vi "PRINCIPAL.vi"() -> ()   [LabVIEW 2019]
uses:
  <vilib>/Analysis/baseanly.llb/Real Dot Product.vi
  <vilib>/Analysis/baseanly.llb/A x Vector.vi
  <vilib>/addons/control/pid/pid.llb/PID (DBL).vi
  <vilib>/Analysis/NI_AALBase.lvlib
  <vilib>/addons/control/pid/NI_PID_pid.lvlib
panel:
  out "FT":picture
  in  "LAZO CERRADO":bool
  in  "setpoint":dbl format="%.2f"
  out "GRAFICA":cluster{"U(t)":dbl, "Y(t)":dbl, dbl}(graph)
  out "Y(t)":dbl format="%.2f"
  out "U(t)":dbl
  in  "Retardo":dbl min=0.0 format="%#_3g"
  in  "Denominador":dbl[](array[numeric])
  in  "Numerador":dbl[](array[numeric])=[0.0, 2.0, 1.0]
  # "LAZO ABIERTO"
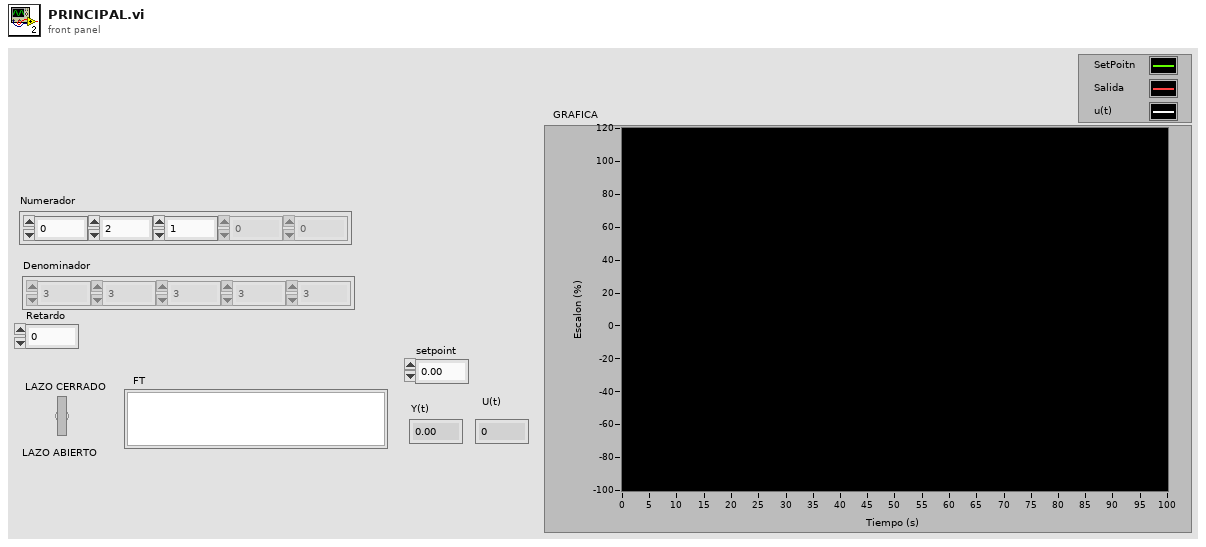
[diagram p1: front panel]
types:
  T1 = typedef "NI_Matrix.lvlib/RealMatrix.ctl" = dbl[][]
  T2 = cluster{"proportional gain (Kc)":dbl, "integral time (Ti, min)":dbl, "derivative time (Td, min)":dbl}
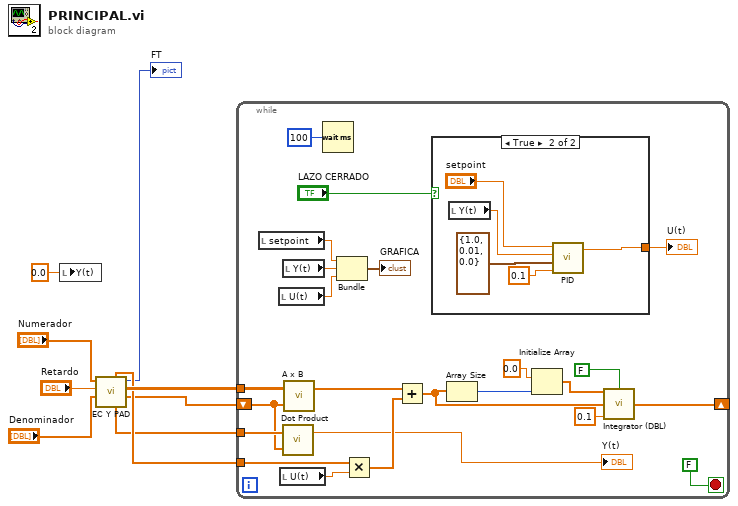
[diagram p0: block diagram]
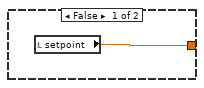
[diagram p2: hidden frame]
diagram:
  n1 = local write "Y(t)"(0.0 ("Y(t)")) -> ()
  n2 = call "EC Y PAD.vi"("Denominador"="Denominador", "Retardo"="Retardo", "Numerador"="Numerador") -> ("Array"=w7:dbl[], "A"=w9:T1, "FT"=→"FT":picture, "C"=w6:dbl[], "B"=w8:dbl[])  [unwired: 4 in]
  n3 = while {
    tunnel: w9 -> [w31]
    tunnel: w8 -> [w30]
    tunnel: w6 -> [w27]
    shift-right: [w19] -> _
    shift-left: w7 -> [w26]
    stop <- FALSE stop-if-true
    n4 = local read "setpoint"() -> (w12:dbl)
    n5 = local read "U(t)"() -> (w15:dbl)
    n6 = local read "U(t)"() -> (w17:dbl)
    n7 = local read "Y(t)"() -> (w13:dbl)
    n8 = call-poly <vilib>:"Dot Product.vi"("Y Vector"=w26, "X Vector"=w27) -> ("X * Y"=→"Y(t)":dbl)  [unwired: 1 out]
    n9 = call-poly <vilib>:"A x B.vi"("Vector"=w26, "A"=w31) -> ("A x Vector"=w29:dbl[])  [unwired: 1 out]
    n10 = Wait (ms)(milliseconds to wait=u32 100) -> ()  [unwired: 1 out]
    n11 = Bundle("setpoint"=w12, "Y(t)"=w13, "U(t)"=w15) -> (→"GRAFICA":cluster{"setpoint":dbl, "Y(t)":dbl, " U(t)":dbl})  [unwired: 1 in]
    n12 = Multiply(x=w30, y=w17) -> (x*y=w28:dbl[])
    n13 = Add ("Add.vi")(x=w29, y=w28) -> (x+y=w23:dbl[])
    n14 = case shown="True" "LAZO CERRADO" {
      tunnel: [w33 w35] -> w11
      frame False {
        n15 = local read "setpoint"() -> (w33:dbl)
      }
      frame True {
        n16 = local read "Y(t)"() -> (w37:dbl)
        n17 = call-poly <vilib>:"PID.vi"("dt (s)"=0.1, "PID gains"=T2 {"proportional gain (Kc)"=1.0, "integral time (Ti, min)"=0.01, "derivative time (Td, min)"=0.0}, "process variable"=w37, "setpoint"="setpoint") -> ("output"=w35:dbl)  [unwired: 6 in, 1 out]
      }
    }
    "U(t)" <- w11
    n18 = Array Size(array=w23) -> (size(s)=w22:i32)
    n19 = Initialize Array(0.0 ("element"), w22) -> (w20:dbl[])
    n20 = call "Integrator (DBL).vi"("initial condition"=w20, "initialize"=FALSE, "input point"=w23, "dt"=0.1) -> ("output"=w19:dbl[])  [unwired: 11 in]
  }
